vi "Division.vi"(0 "x":dbl, 5 "y":dbl, 11 "error in (no error)":errorcluster) -> (4 "quotient":dbl, 15 "error out":errorcluster)   [LabVIEW 2015]
uses:
  Exceptions/Exception Division By Zero/Exception Division By Zero.lvclass
  <userlib>/LV Exceptions v1/Exception/Exception.lvclass/Exception.ctl
  <vilib>/Utility/error.llb/Trim Whitespace.vi
  <userlib>/LV Exceptions v1/Exception/Exception.lvclass
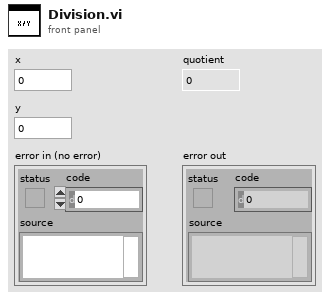
[diagram p1: front panel]
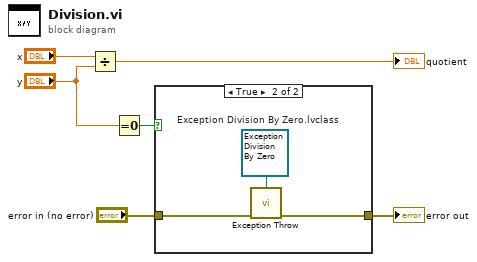
[diagram p0: block diagram]
diagram:
  n1 = Divide(x="x", y="y") -> (x/y=→"quotient":dbl)
  n2 = Equal To 0?(x="y") -> (x = 0?=w3:bool)
  n3 = case shown="True" w3 {
    tunnel: "error in (no error)" -> [w7 w9]
    tunnel: [w7 w8] -> w1
    frame False {
    }
    frame True {
      w10 = refnum<class "Exception Division By Zero.lvclass"> refnum  # Exception Division By Zero.lvclass
      n4 = call <userlib>:"Exception Throw.vi"("Exception in"=w10, "error in (no error)"=w9) -> ("error out"=w8:errorcluster)  [unwired: 13 in]
    }
  }
  "error out" <- w1
